vi "VFH-read_file-libreVNA.vi"(8 "error in":errorcluster, 10 "file path (dialog if empty)":path=path "C:/projects/Universitet/Master/code/data/1_Intial_measurements/cap.s1p") -> (0 "error out":errorcluster, 2 "output cluster":T1)   [LabVIEW 2020, in "VFH-VNA_File_Handler.lvlib"]
uses:
  VFH-file_cluster-NanoVNA.ctl
  VFH-VNA_File_Handler.lvlib
panel:
  out "string array 2":string[][](array[string])
  out "string array":string[](array[string])
  out "after substring":string
  out "text":string
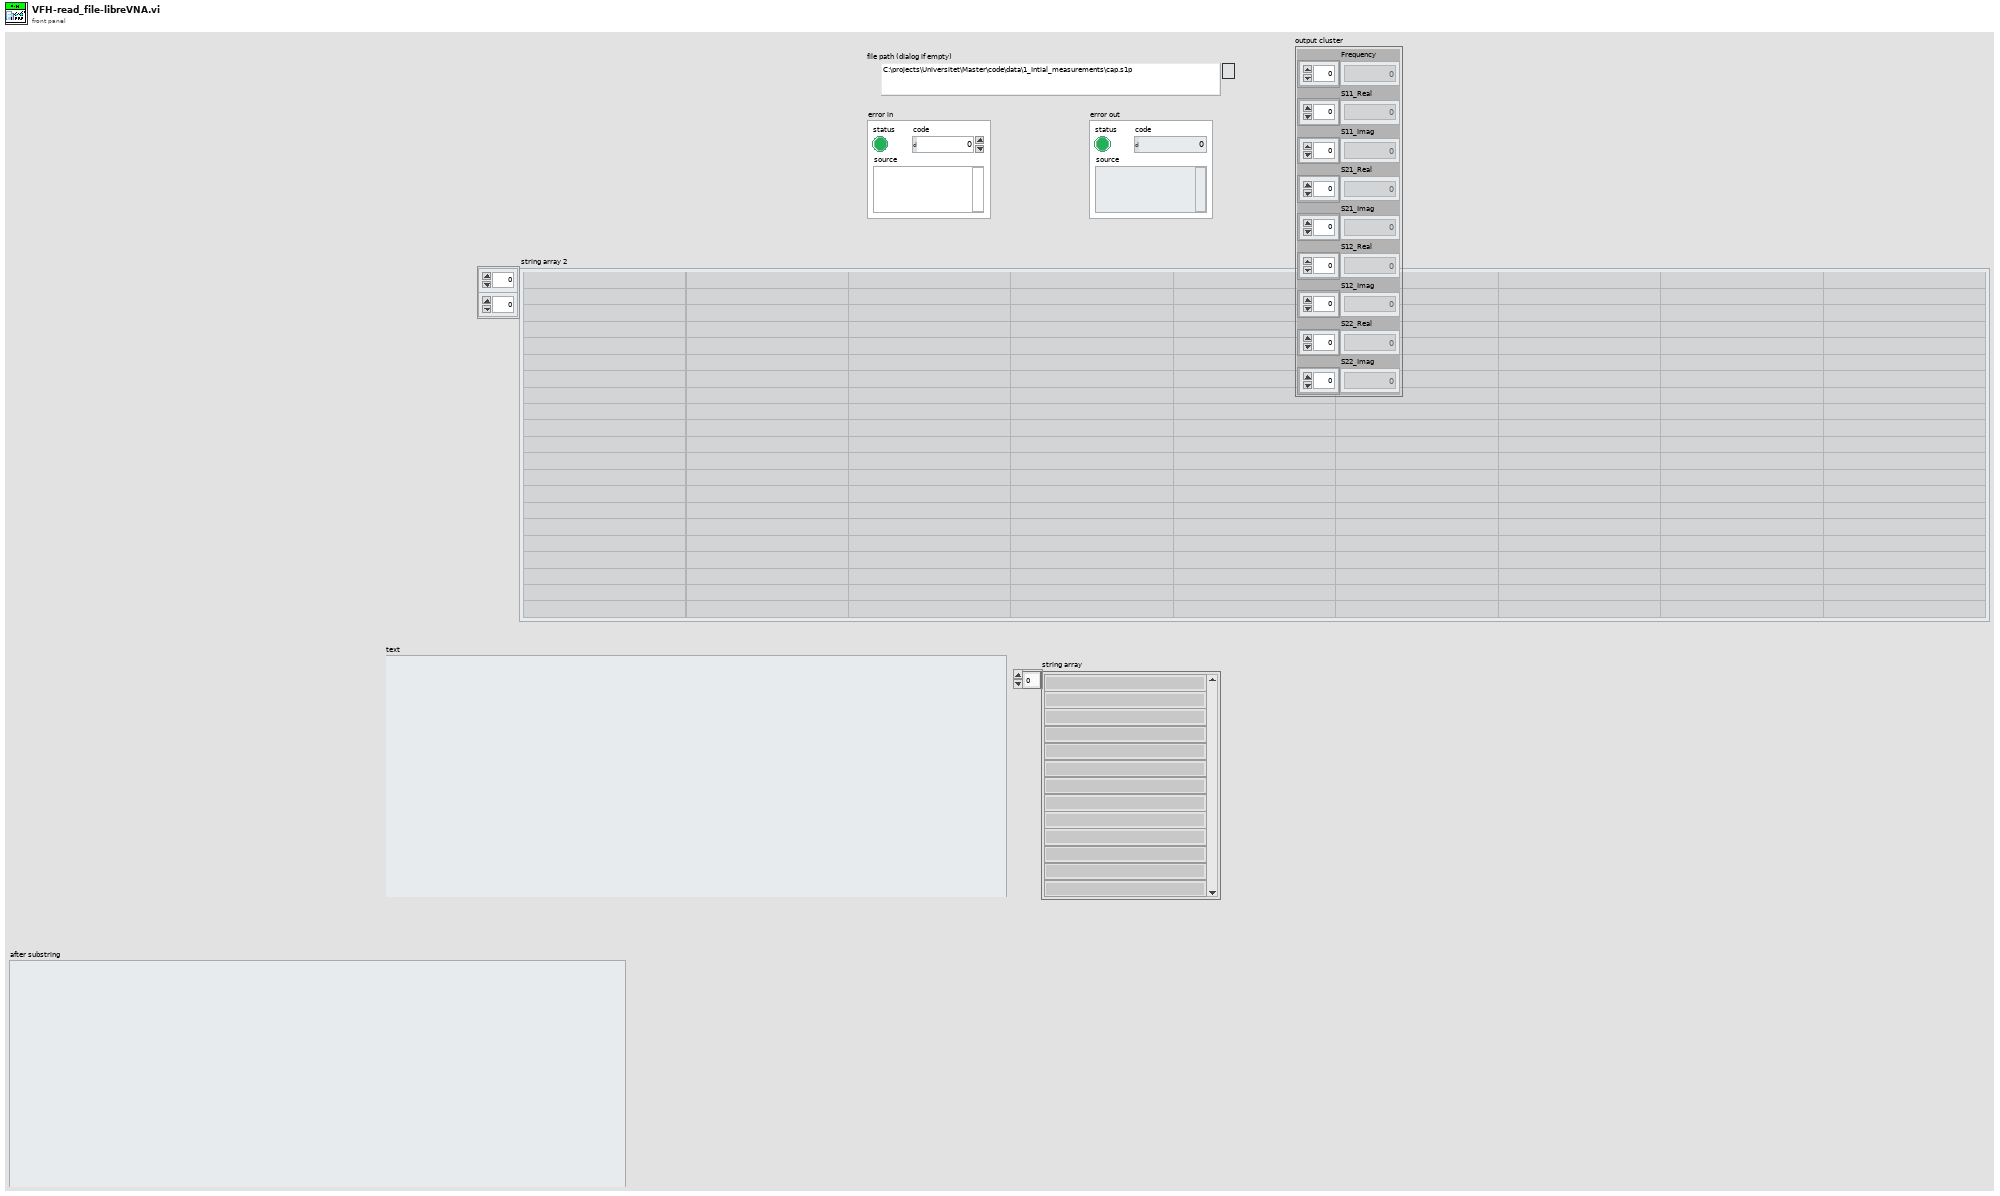
[diagram p1: front panel]
types:
  T1 = typedef "VFH-VNA_File_Handler.lvlib/VFH-file_cluster-NanoVNA.ctl" = cluster{"Frequency":dbl[], "S11_Real":dbl[], "S11_Imag":dbl[], "S21_Real":dbl[], "S21_Imag":dbl[], "S12_Real":dbl[], "S12_Imag":dbl[], "S22_Real":dbl[], "S22_Imag":dbl[]}
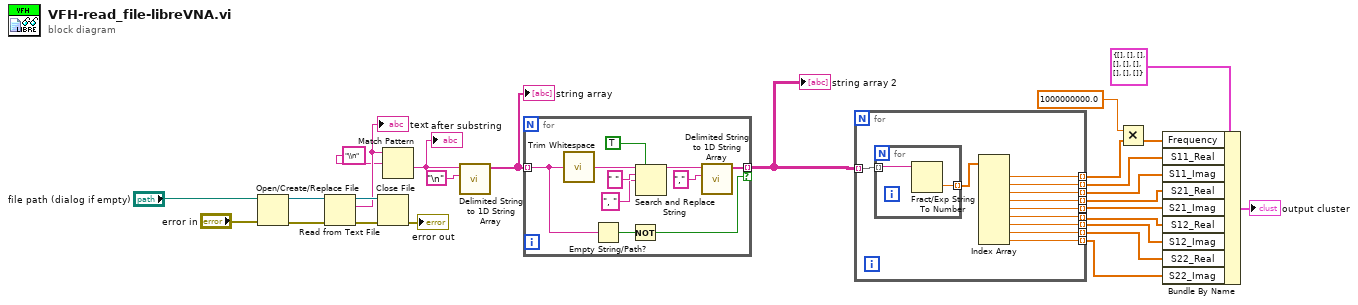
[diagram p0: block diagram]
diagram:
  n1 = Open/Create/Replace File(file path (use dialog)="file path (dialog if empty)", error in="error in") -> (refnum out=w26:refnum<file>, error out=w23:errorcluster)  [unwired: 4 in, 1 out]
  n2 = Read from Text File(file (use dialog)=w26, error in=w23) -> (refnum out=w25:refnum<file>, text=w21:string, error out=w24:errorcluster)  [unwired: 2 in, 1 out]
  "text" <- w21
  n3 = Close File(refnum=w25, error in=w24) -> (error out=→"error out":errorcluster)  [unwired: 1 out]
  n4 = Match Pattern(string=w21, regular expression="\\n" ("search string/char (-)")) -> (after substring=w17:string)  [unwired: 1 in, 3 out]
  "after substring" <- w17
  n5 = call <vilib>:"Delimited String to 1D String Array.vi"("delimiter"="\n", "delimited string"=w17) -> ("string array"=w18:string[])  [unwired: 9 in]
  "string array" <- w18
  n6 = for {
    tunnel: w18 -> [w28] mode=indexing
    tunnel: [w36] -> w16 mode=indexing if=w27
    n7 = call <vilib>:"Trim Whitespace.vi"("string"=w28) -> ("trimmed string"=w35:string)  [unwired: 1 in]
    n8 = Empty String/Path?(string/path=w28) -> (empty?=w29:bool)
    n9 = Not(x=w29) -> (.not. x?=w27:bool)
    n10 = Search and Replace String(replace all?=TRUE ("replace all? (F)"), input string=w35, search string=" ", replace string=", " ("replace string (\"\")")) -> (result string=w30:string)  [unwired: 4 in, 3 out]
    n11 = call <vilib>:"Delimited String to 1D String Array.vi"("delimiter"=",", "delimited string"=w30) -> ("string array"=w36:string[])  [unwired: 9 in]
  }
  "string array 2" <- w16
  n12 = for {
    tunnel: w16 -> [w47] mode=indexing
    tunnel: [w45] -> w15 mode=indexing
    tunnel: [w44] -> w14 mode=indexing
    tunnel: [w43] -> w13 mode=indexing
    tunnel: [w42] -> w12 mode=indexing
    tunnel: [w41] -> w11 mode=indexing
    tunnel: [w40] -> w10 mode=indexing
    tunnel: [w39] -> w9 mode=indexing
    tunnel: [w38] -> w8 mode=indexing
    tunnel: [w37] -> w7 mode=indexing
    n13 = for {
      tunnel: w47 -> [w49] mode=indexing
      tunnel: [w48] -> w46 mode=indexing
      n14 = Fract/Exp String To Number(string=w49) -> (number=w48:dbl)  [unwired: 3 in, 1 out]
    }
    n15 = Index Array(array=w46) -> (element #1=w45:dbl, element #2=w44:dbl, element #3=w43:dbl, element #4=w42:dbl, element #5=w41:dbl, element #6=w40:dbl, element #7=w39:dbl, element #8=w38:dbl, element #9=w37:dbl)  [unwired: 9 in]
  }
  n16 = Multiply(x=1000000000.0 ("element"), y=w15) -> (x*y=w2:dbl[])
  n17 = Bundle By Name(cluster=T1 {"Frequency"=[], "S11_Real"=[], "S11_Imag"=[], "S21_Real"=[], "S21_Imag"=[], "S12_Real"=[], "S12_Imag"=[], "S22_Real"=[], "S22_Imag"=[]} ("output cluster"), "Frequency"=w2, "S11_Real"=w14, "S11_Imag"=w13, "S21_Real"=w12, "S21_Imag"=w11, "S12_Real"=w10, "S12_Imag"=w9, "S22_Real"=w8, "S22_Imag"=w7) -> (→"output cluster":T1)
